vi "Clip &Lvdt Data.vi"(0 "Pokayoka":T2, 2 "Result Lvdt in":T1) -> (7 "Clip Status":string, 8 "Screw Height Status":string)   [LabVIEW 2015]
uses:
  Galobal variable_TI.vi
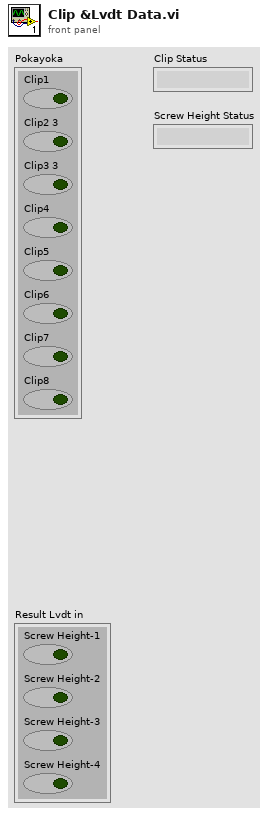
[diagram p1: front panel]
types:
  T1 = cluster{"Screw Height-1":bool, "Screw Height-2":bool, "Screw Height-3":bool, "Screw Height-4":bool}
  T2 = cluster{"Clip1":bool, "Clip2 3":bool, "Clip3 3":bool, "Clip4":bool, "Clip5":bool, "Clip6":bool, "Clip7":bool, "Clip8":bool}
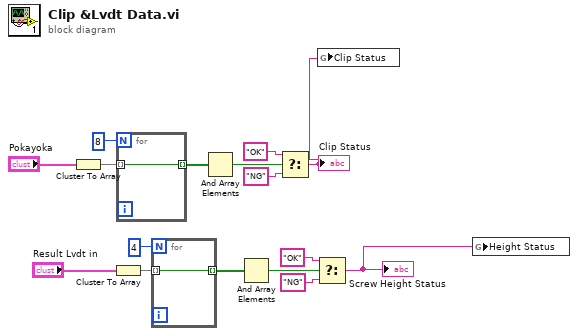
[diagram p0: block diagram]
diagram:
  n1 = Cluster To Array(cluster="Pokayoka") -> (array=w15:bool[])
  n2 = Cluster To Array(cluster="Result Lvdt in") -> (array=w5:bool[])
  n3 = for {
    N: 8 -> [_]
    tunnel: w15 -> [w17] mode=indexing
    tunnel: [w17] -> w13 mode=indexing
  }
  n4 = for {
    N: 4 -> [_]
    tunnel: w5 -> [w18] mode=indexing
    tunnel: [w18] -> w4 mode=indexing
  }
  n5 = And Array Elements(Boolean array=w13) -> (logical AND=w12:bool)
  n6 = And Array Elements(Boolean array=w4) -> (logical AND=w6:bool)
  n7 = Select(t="OK" ("Screw -FL"), s=w12, f="NG" ("Screw -FL")) -> (s? t:f=w2:string)
  "Clip Status" <- w2
  n8 = Select(t="OK" ("Screw -FL"), s=w6, f="NG" ("Screw -FL")) -> (s? t:f=w1:string)
  "Screw Height Status" <- w1
  n9 = global write "Galobal variable_TI.vi" "Clip Status"(w2) -> ()
  n10 = global write "Galobal variable_TI.vi" "Height Status"(w1) -> ()
